vi "AuMT8852B Output Power Test Configuration.vi"(5 "Settings":T1={"Hop mode"=enum."Defined", "Low frequency selection"=enum."Use low frequency", "Medium frequency selection"=enum."Use medium frequency", "High frequency selection"=enum."Use high frequency", "Low TX frequency"=2402.0, "Medium TX frequency"=2441.0, "High TX frequency"=2480.0, "Number of packets"=10, "Packet type"=enum."Longest supported", "Test control"=enum."Loopback", "Average power high limit"=20.0, "Average power low limit"=-6.0, "Peak power limit"=23.0, "Hop selection"=enum."Test with hopping on", "Low RX frequency"=2402.0, "Medium RX frequency"=2441.0, "High RX frequency"=2480.0} {"Peak power limit" format="%.1f"; "Average power low limit" format="%.1f"; "Average power high limit" format="%.1f"}, 7 "Set/Get (Set)":enum16{"Set", "Get"}(ring), 8 "error in (no error)":errorcluster, 9 "Frequency units (MHz)":T2=enum."MHz", 10 "Script (3)":i32=3, 11 "VISA session":refnum<visa-resource-name>) -> (0 "error out":errorcluster, 2 "error code":i32, 3 "VISA session out":refnum<visa-resource-name>, 4 "Settings out":T1={"Hop mode"=enum."Defined", "Low frequency selection"=enum."Use low frequency", "Medium frequency selection"=enum."Use medium frequency", "High frequency selection"=enum."Use high frequency", "Low TX frequency"=0.0, "Medium TX frequency"=0.0, "High TX frequency"=0.0, "Number of packets"=0, "Packet type"=enum."Longest supported", "Test control"=enum."Loopback", "Average power high limit"=0.0, "Average power low limit"=0.0, "Peak power limit"=0.0, "Hop selection"=enum."Test with hopping on", "Low RX frequency"=2402.0, "Medium RX frequency"=2441.0, "High RX frequency"=2480.0} {"Peak power limit" format="%.1f"; "Average power low limit" format="%.1f"; "Average power high limit" format="%.1f"})   [LabVIEW 2017]
doc: "Anritsu MT8852B Bluetooth Tester\n\nConfigures the instrument for the Output Power test.\n\nINPUTS\nSet/Get - whether the values are being sent to or retrieved from the instrument.\nScript - which of the stored scripts (1-10) will be queried or configured. Scripts 1 and 2 are read-only.\nFrequency units - whether the low, medium, and high frequencies are expressed as a channel or as a frequency in Hz, kHz, MHz, or GHz.\nSettings - parameters of the test to be written.\n\nOUTPUTS\nSettings out - current parameters of the test."
uses:
  <instrlib>/aumt8852B/General/Utilities/MT8850 Frequency Units.ctl
  <instrlib>/aumt8852B/General/Utilities/MT8850 Test Parameters.ctl
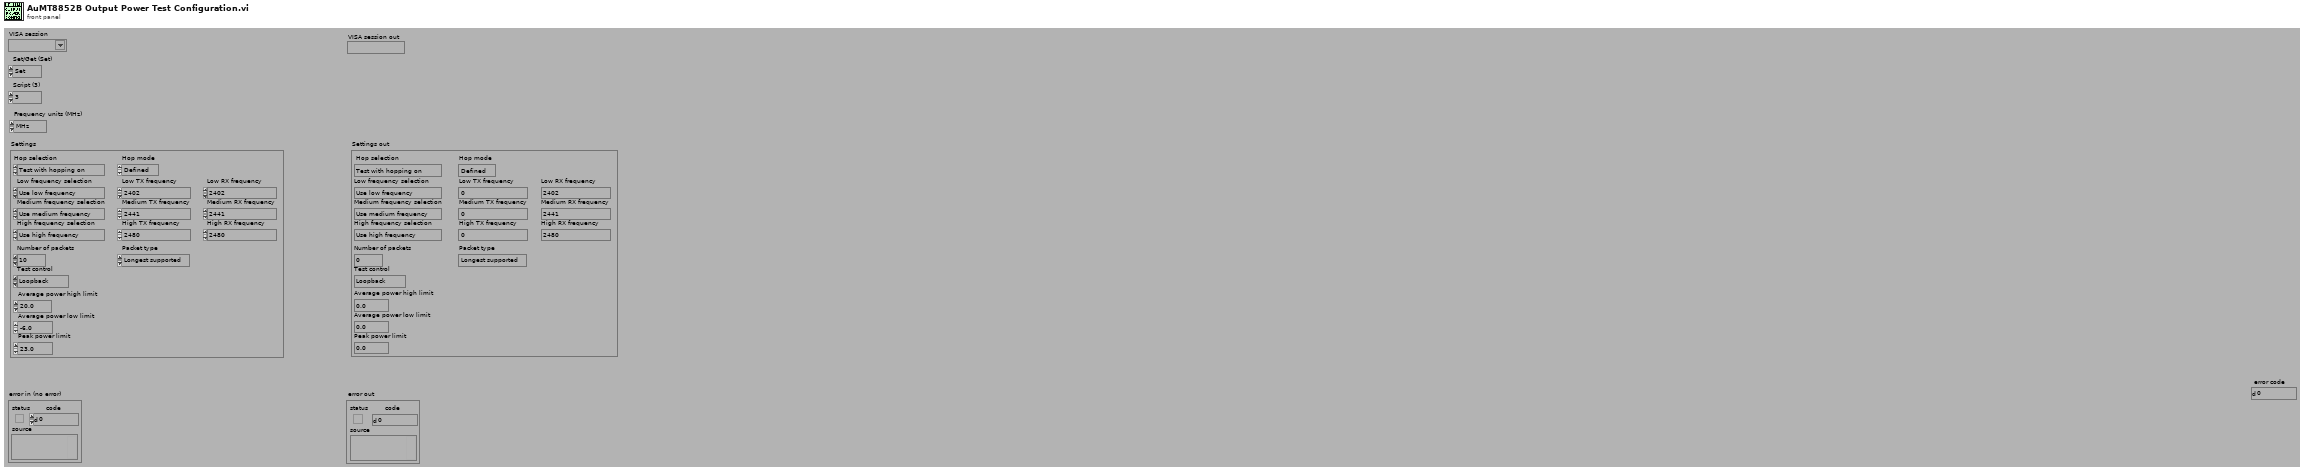
[diagram p1: front panel]
types:
  T1 = cluster{"Hop mode":enum16{"All", "Any", "Defined"}, "Low frequency selection":enum16{"Don't use low frequency", "Use low frequency"}, "Medium frequency selection":enum16{"Don't use medium frequency", "Use medium frequency"}, "High frequency selection":enum16{"Don't use high frequency", "Use high frequency"}, "Low TX frequency":dbl, "Medium TX frequency":dbl, "High TX frequency":dbl, "Number of packets":i32, "Packet type":enum16{"Longest supported", "DH5", "DH3", "DH1"}, "Test control":enum16{"Loopback", "TX test"}, "Average power high limit":dbl, "Average power low limit":dbl, "Peak power limit":dbl, "Hop selection":enum16{"Test with hopping on", "Test with hopping off", "Test with hopping on and off"}, "Low RX frequency":dbl, "Medium RX frequency":dbl, "High RX frequency":dbl}
  T2 = typedef "MT8850 Frequency Units.ctl" = enum16{"Channel", "Hz", "kHz", "MHz", "GHz"}
  T3 = typedef "MT8850 Test Parameters.ctl" = enum16{"Use low frequency", "Use medium frequency", "Use high frequency", "Low TX frequency", "Low RX frquency", "Medium TX frequency", "Medium RX frequency", "High TX frequency", "High RX frequency", "Number of packets", "Average high limit", "Average low limit", "Peak power limit", "Max power step limit", "Min power step limit", "f1 average minimum", "f1 average maximum", "f2 maximum", "f1/f2 average maximum", "Hop selection", "Use DH1 packets", "Use DH3 packets", "Use DH5 packets", "1 slot packet drift limit", "3 slot packet drift limit", "5 slot packet drift limit", "Drift rate limit", "TX power level", "Frequency offset", "Symbol timing", "Modulation index", "BER limit", "FER limit", "Use averaging high limit", "Use averaging low limit", "Use peak power limit", "Packet type", "Test control", "Use max power step limit", "Use min power step limit", "Number of cycles", "Use f1 average maximum", "Use f1 average minimum", "Use f2 maximum", "Use f1/f2 average maximum", "Hop mode", "Maximum negative limit", "Maximum positive limit", "Use maximum negative limit", "Use maximum positive limit", "Use 1 slot packet drift limit", "Use 3 slot packet drift limit", "Use 5 slot packet drift limit", "Use drift rate limit", "Use BER limit", "Use FER limit", "Use dirty parameter table", "Use null packet drift limit", "Null packet drift limit", "Minimum power", "Power delay", "Packet count", "Payload toggle", "Output power level", "2DHX packet type", "3DHX packet type", "Number of blocks", "TX and RX low frequency", "TX and RX medium frequency", "TX and RX high frequency", "TX frequency", "RX frequency", "Threshold bit count", "Total test bit count", "Number of bits", "PDPSK to PGFSK lower limit", "PDPSK to PGFSK upper limit", "Initial frequency error upper limit", "Initial frequency error lower limit", "Frequency error upper limit", "Frequency error lower limit", "Block frequency error upper limit", "Block frequency error lower limit", "2Mbs RMS DEVM limit", "3Mbs RMS DEVM limit", "2Mbs Peak DEVM limit", "3Mbs Peak DEVM limit", "2Mbs 99% packets DEVM limit", "3Mbs 99% packets DEVM limit", "Percentage of no error packets limit", "Threshold error limit", "Total test error limit"}
  T4 = enum16{"Simulate", "Range check", "Cache", "Query instrument status"}
  T5 = enum16{"Output power", "Power control", "Modulation characteristics", "Initial carrier", "Carrier drift", "Single slot sensitivity", "Multiple slot sensitivity", "Maximum input power"}
  T6 = enum16{"Don't use high frequency", "Use high frequency"}
  T7 = enum16{"Don't use medium frequency", "Use medium frequency"}
  T8 = enum16{"Don't use low frequency", "Use low frequency"}
  T9 = enum16{"Test with hopping on", "Test with hopping off", "Test with hopping on and off"}
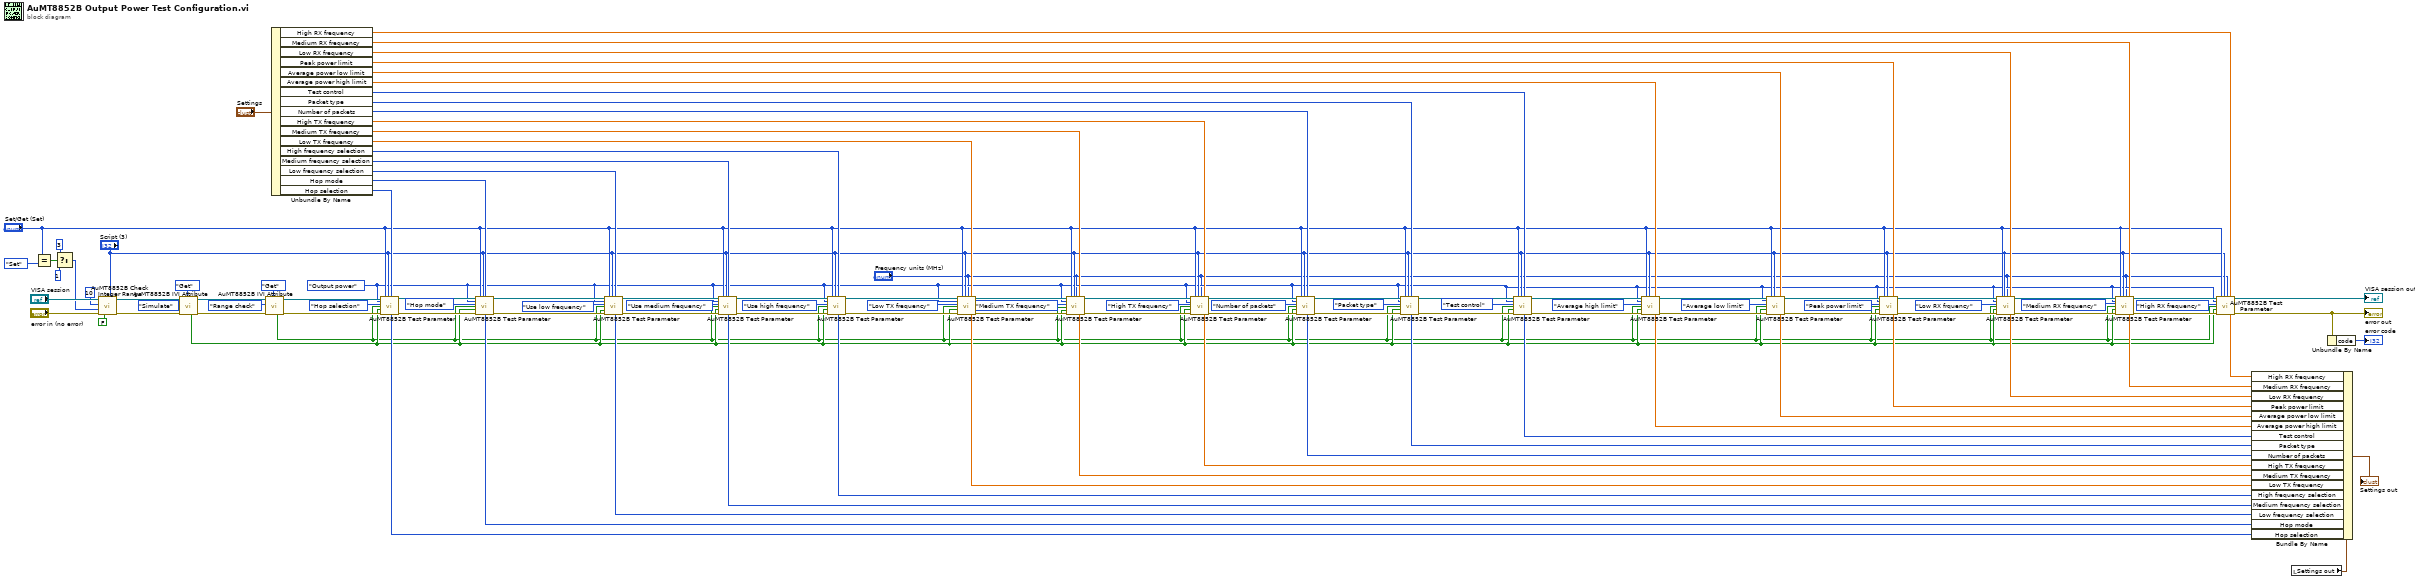
[diagram p0: block diagram]
diagram:
  w2 = T5."Output power" ("Test (Output Power)")
  n1 = Equal?(x="Set/Get (Set)", y=enum16{"Set", "Get"}."Set") -> (x = y?=w111:bool)
  n2 = Select(t=3, s=w111, f=1) -> (s? t:f=w107:i32)
  n3 = call <instrlib>:"AuMT8852B Check Integer Range.vi"("Value (0)"="Script (3)", "Check IVI flag first? (T)"=FALSE, "error in (no error)"="error in (no error)", "Lower limit (-1)"=w107, "Upper limit (1)"=10, "VISA session"="VISA session") -> ("error out"=w105:errorcluster, "VISA session out"=w106:refnum<visa-resource-name>)  [unwired: 4 in]
  n4 = call <instrlib>:"AuMT8852B IVI Attribute.vi"("Set/Get (Set)"=enum16{"Set", "Get"}."Get", "error in (no error)"=w105, "Flag (Simulate)"=T4."Simulate", "VISA session"=w106) -> ("error out"=w85:errorcluster, "VISA session out"=w86:refnum<visa-resource-name>, "Value out"=w12:bool)  [unwired: 5 in]
  n5 = call <instrlib>:"AuMT8852B IVI Attribute.vi"("Set/Get (Set)"=enum16{"Set", "Get"}."Get", "error in (no error)"=w85, "Flag (Simulate)"=T4."Range check", "VISA session"=w86) -> ("error out"=w38:errorcluster, "VISA session out"=w36:refnum<visa-resource-name>, "Value out"=w11:bool)  [unwired: 5 in]
  n6 = Unbundle By Name("Settings") -> ("High RX frequency"=w5:dbl, "Medium RX frequency"=w6:dbl, "Low RX frequency"=w7:dbl, "Peak power limit"=w72:dbl, "Average power low limit"=w73:dbl, "Average power high limit"=w74:dbl, "Test control"=w47:enum16{"Loopback", "TX test"}, "Packet type"=w48:enum16{"Longest supported", "DH5", "DH3", "DH1"}, "Number of packets"=w75:i32, "High TX frequency"=w76:dbl, "Medium TX frequency"=w77:dbl, "Low TX frequency"=w78:dbl, "High frequency selection"=w79:T6, "Medium frequency selection"=w80:T7, "Low frequency selection"=w81:T8, "Hop mode"=w58:enum16{"All", "Any", "Defined"}, "Hop selection"=w33:T9)
  n7 = call <instrlib>:"AuMT8852B Test Parameter.vi"("VISA session"=w36, "Test (Output power)"=w2, "Parameter (Use low frequency)"=MT8850_Test_Parameters."Hop selection", "Range check? (F)"=w11, "Simulate? (F)"=w12, "error in (no error)"=w38, "Set/Get (Set)"="Set/Get (Set)", "Script (3)"="Script (3)", "Integer value (0)"=w33) -> ("Integer value out"=w32:i32, "VISA session out"=w35:refnum<visa-resource-name>, "error out"=w37:errorcluster)  [unwired: 7 in, 1 out]
  n8 = call <instrlib>:"AuMT8852B Test Parameter.vi"("VISA session"=w35, "Test (Output power)"=w2, "Parameter (Use low frequency)"=MT8850_Test_Parameters."Hop mode", "Range check? (F)"=w11, "Simulate? (F)"=w12, "error in (no error)"=w37, "Set/Get (Set)"="Set/Get (Set)", "Script (3)"="Script (3)", "Integer value (0)"=w58) -> ("Integer value out"=w57:i32, "VISA session out"=w61:refnum<visa-resource-name>, "error out"=w60:errorcluster)  [unwired: 7 in, 1 out]
  n9 = call <instrlib>:"AuMT8852B Test Parameter.vi"("VISA session"=w61, "Test (Output power)"=w2, "Parameter (Use low frequency)"=MT8850_Test_Parameters."Use low frequency", "Range check? (F)"=w11, "Simulate? (F)"=w12, "error in (no error)"=w60, "Set/Get (Set)"="Set/Get (Set)", "Script (3)"="Script (3)", "Integer value (0)"=w81) -> ("Integer value out"=w62:i32, "VISA session out"=w44:refnum<visa-resource-name>, "error out"=w43:errorcluster)  [unwired: 7 in, 1 out]
  n10 = call <instrlib>:"AuMT8852B Test Parameter.vi"("VISA session"=w44, "Test (Output power)"=w2, "Parameter (Use low frequency)"=MT8850_Test_Parameters."Use medium frequency", "Range check? (F)"=w11, "Simulate? (F)"=w12, "error in (no error)"=w43, "Set/Get (Set)"="Set/Get (Set)", "Script (3)"="Script (3)", "Integer value (0)"=w80) -> ("Integer value out"=w63:i32, "VISA session out"=w42:refnum<visa-resource-name>, "error out"=w41:errorcluster)  [unwired: 7 in, 1 out]
  n11 = call <instrlib>:"AuMT8852B Test Parameter.vi"("VISA session"=w42, "Test (Output power)"=w2, "Parameter (Use low frequency)"=MT8850_Test_Parameters."Use high frequency", "Range check? (F)"=w11, "Simulate? (F)"=w12, "error in (no error)"=w41, "Set/Get (Set)"="Set/Get (Set)", "Script (3)"="Script (3)", "Integer value (0)"=w79) -> ("Integer value out"=w64:i32, "VISA session out"=w101:refnum<visa-resource-name>, "error out"=w100:errorcluster)  [unwired: 7 in, 1 out]
  n12 = call <instrlib>:"AuMT8852B Test Parameter.vi"("VISA session"=w101, "Test (Output power)"=w2, "Parameter (Use low frequency)"=MT8850_Test_Parameters."Low TX frequency", "Range check? (F)"=w11, "Simulate? (F)"=w12, "error in (no error)"=w100, "Set/Get (Set)"="Set/Get (Set)", "Script (3)"="Script (3)", "Integer value (0)"="Frequency units (MHz)", "Float value (0)"=w78) -> ("Float value out"=w65:dbl, "VISA session out"=w99:refnum<visa-resource-name>, "error out"=w98:errorcluster)  [unwired: 6 in, 1 out]
  n13 = call <instrlib>:"AuMT8852B Test Parameter.vi"("VISA session"=w99, "Test (Output power)"=w2, "Parameter (Use low frequency)"=MT8850_Test_Parameters."Medium TX frequency", "Range check? (F)"=w11, "Simulate? (F)"=w12, "error in (no error)"=w98, "Set/Get (Set)"="Set/Get (Set)", "Script (3)"="Script (3)", "Integer value (0)"="Frequency units (MHz)", "Float value (0)"=w77) -> ("Float value out"=w66:dbl, "VISA session out"=w97:refnum<visa-resource-name>, "error out"=w96:errorcluster)  [unwired: 6 in, 1 out]
  n14 = call <instrlib>:"AuMT8852B Test Parameter.vi"("VISA session"=w97, "Test (Output power)"=w2, "Parameter (Use low frequency)"=MT8850_Test_Parameters."High TX frequency", "Range check? (F)"=w11, "Simulate? (F)"=w12, "error in (no error)"=w96, "Set/Get (Set)"="Set/Get (Set)", "Script (3)"="Script (3)", "Integer value (0)"="Frequency units (MHz)", "Float value (0)"=w76) -> ("Float value out"=w67:dbl, "VISA session out"=w95:refnum<visa-resource-name>, "error out"=w94:errorcluster)  [unwired: 6 in, 1 out]
  n15 = call <instrlib>:"AuMT8852B Test Parameter.vi"("VISA session"=w95, "Test (Output power)"=w2, "Parameter (Use low frequency)"=MT8850_Test_Parameters."Number of packets", "Range check? (F)"=w11, "Simulate? (F)"=w12, "error in (no error)"=w94, "Set/Get (Set)"="Set/Get (Set)", "Script (3)"="Script (3)", "Integer value (0)"=w75) -> ("Integer value out"=w68:i32, "VISA session out"=w56:refnum<visa-resource-name>, "error out"=w55:errorcluster)  [unwired: 7 in, 1 out]
  n16 = call <instrlib>:"AuMT8852B Test Parameter.vi"("VISA session"=w56, "Test (Output power)"=w2, "Parameter (Use low frequency)"=MT8850_Test_Parameters."Packet type", "Range check? (F)"=w11, "Simulate? (F)"=w12, "error in (no error)"=w55, "Set/Get (Set)"="Set/Get (Set)", "Script (3)"="Script (3)", "Integer value (0)"=w48) -> ("Integer value out"=w50:i32, "VISA session out"=w53:refnum<visa-resource-name>, "error out"=w52:errorcluster)  [unwired: 7 in, 1 out]
  n17 = call <instrlib>:"AuMT8852B Test Parameter.vi"("VISA session"=w53, "Test (Output power)"=w2, "Parameter (Use low frequency)"=MT8850_Test_Parameters."Test control", "Range check? (F)"=w11, "Simulate? (F)"=w12, "error in (no error)"=w52, "Set/Get (Set)"="Set/Get (Set)", "Script (3)"="Script (3)", "Integer value (0)"=w47) -> ("Integer value out"=w49:i32, "VISA session out"=w30:refnum<visa-resource-name>, "error out"=w31:errorcluster)  [unwired: 7 in, 1 out]
  n18 = call <instrlib>:"AuMT8852B Test Parameter.vi"("VISA session"=w30, "Test (Output power)"=w2, "Parameter (Use low frequency)"=MT8850_Test_Parameters."Average high limit", "Range check? (F)"=w11, "Simulate? (F)"=w12, "error in (no error)"=w31, "Set/Get (Set)"="Set/Get (Set)", "Script (3)"="Script (3)", "Float value (0)"=w74) -> ("Float value out"=w69:dbl, "VISA session out"=w28:refnum<visa-resource-name>, "error out"=w29:errorcluster)  [unwired: 7 in, 1 out]
  n19 = call <instrlib>:"AuMT8852B Test Parameter.vi"("VISA session"=w28, "Test (Output power)"=w2, "Parameter (Use low frequency)"=MT8850_Test_Parameters."Average low limit", "Range check? (F)"=w11, "Simulate? (F)"=w12, "error in (no error)"=w29, "Set/Get (Set)"="Set/Get (Set)", "Script (3)"="Script (3)", "Float value (0)"=w73) -> ("Float value out"=w70:dbl, "VISA session out"=w26:refnum<visa-resource-name>, "error out"=w27:errorcluster)  [unwired: 7 in, 1 out]
  n20 = call <instrlib>:"AuMT8852B Test Parameter.vi"("VISA session"=w26, "Test (Output power)"=w2, "Parameter (Use low frequency)"=MT8850_Test_Parameters."Peak power limit", "Range check? (F)"=w11, "Simulate? (F)"=w12, "error in (no error)"=w27, "Set/Get (Set)"="Set/Get (Set)", "Script (3)"="Script (3)", "Float value (0)"=w72) -> ("Float value out"=w71:dbl, "VISA session out"=w22:refnum<visa-resource-name>, "error out"=w23:errorcluster)  [unwired: 7 in, 1 out]
  n21 = call <instrlib>:"AuMT8852B Test Parameter.vi"("VISA session"=w22, "Test (Output power)"=w2, "Parameter (Use low frequency)"=MT8850_Test_Parameters."Low RX frquency", "Range check? (F)"=w11, "Simulate? (F)"=w12, "error in (no error)"=w23, "Set/Get (Set)"="Set/Get (Set)", "Script (3)"="Script (3)", "Integer value (0)"="Frequency units (MHz)", "Float value (0)"=w7) -> ("Float value out"=w17:dbl, "VISA session out"=w19:refnum<visa-resource-name>, "error out"=w20:errorcluster)  [unwired: 6 in, 1 out]
  n22 = call <instrlib>:"AuMT8852B Test Parameter.vi"("VISA session"=w19, "Test (Output power)"=w2, "Parameter (Use low frequency)"=MT8850_Test_Parameters."Medium RX frequency", "Range check? (F)"=w11, "Simulate? (F)"=w12, "error in (no error)"=w20, "Set/Get (Set)"="Set/Get (Set)", "Script (3)"="Script (3)", "Integer value (0)"="Frequency units (MHz)", "Float value (0)"=w6) -> ("Float value out"=w16:dbl, "VISA session out"=w13:refnum<visa-resource-name>, "error out"=w14:errorcluster)  [unwired: 6 in, 1 out]
  n23 = call <instrlib>:"AuMT8852B Test Parameter.vi"("VISA session"=w13, "Test (Output power)"=w2, "Parameter (Use low frequency)"=MT8850_Test_Parameters."High RX frequency", "Range check? (F)"=w11, "Simulate? (F)"=w12, "error in (no error)"=w14, "Set/Get (Set)"="Set/Get (Set)", "Script (3)"="Script (3)", "Integer value (0)"="Frequency units (MHz)", "Float value (0)"=w5) -> ("Float value out"=w10:dbl, "VISA session out"=→"VISA session out":refnum<visa-resource-name>, "error out"=w9:errorcluster)  [unwired: 6 in, 1 out]
  "error out" <- w9
  n24 = local read "Settings out"() -> (w25:T1)
  n25 = Bundle By Name(cluster=w25, "High RX frequency"=w10, "Medium RX frequency"=w16, "Low RX frequency"=w17, "Peak power limit"=w71, "Average power low limit"=w70, "Average power high limit"=w69, "Test control"=w49, "Packet type"=w50, "Number of packets"=w68, "High TX frequency"=w67, "Medium TX frequency"=w66, "Low TX frequency"=w65, "High frequency selection"=w64, "Medium frequency selection"=w63, "Low frequency selection"=w62, "Hop mode"=w57, "Hop selection"=w32) -> (→"Settings out":T1)
  n26 = Unbundle By Name(w9) -> ("code"=→"error code":i32)
